vi "Editor Message List Creator.vi"(8 "error in (no error)":errorcluster, 10 "Message List":refnum<vi>, 11 "Hierarchy":refnum<vi>) -> (0 "error out":errorcluster, 3 "Message List Elements":T1[](array[typedef]))   [LabVIEW 2020]
doc: "Create Array of Message List Elements from either the Folder Override or from the Application data folder."
uses:
  Controls/Ctl_MessageListElement.ctl
  Sequencer.lvlib
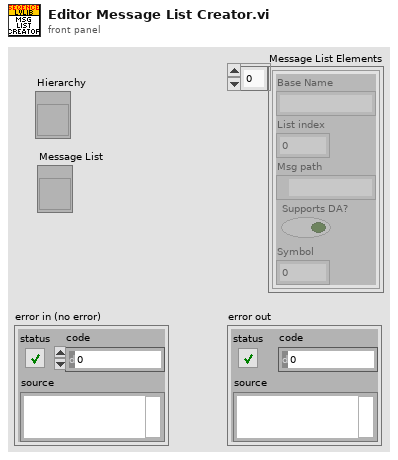
[diagram p1: front panel]
types:
  T1 = typedef "Sequencer.lvlib/Ctl_MessageListElement.ctl" = cluster{"Base Name":string, "List index":i32, "Msg path":path, "Supports DA?":bool, "Symbol":i32}
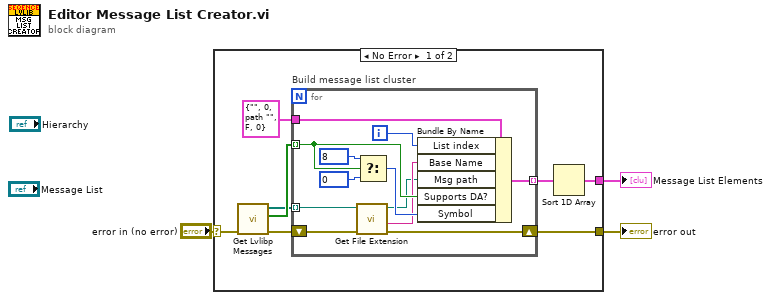
[diagram p0: block diagram]
diagram:
  n1 = case shown="No Error" "error in (no error)" {
    selector: "error in (no error)" -> [w9 w24]
    tunnel: [w10 w24] -> w3
    tunnel: [w8 _] -> w1
    frame No Error {
      n2 = call "Get Lvlibp Messages.vi"("error in (no error)"=w9) -> ("error out"=w11:errorcluster, "Supports Data Access?"=w5:bool[], "Msg Paths"=w4:path[])  [unwired: 7 in, 1 out]
      n3 = for "Build message list cluster" {
        tunnel: w4 -> [w23] mode=indexing
        tunnel: w5 -> [w18] mode=indexing
        shift-right: [w16] -> w10
        shift-left: w11 -> [w20]
        tunnel: T1 {"Base Name"="", "List index"=0, "Msg path"=path "", "Supports DA?"=FALSE, "Symbol"=0} -> [w19]
        tunnel: [w17] -> w7 mode=indexing
        i -> [w14]
        n4 = call <vilib>:"Get File Extension.vi"("error in (no error)"=w20, "file"=w23) -> ("error out"=w16:errorcluster, "filename without extension"=w13:string, "dup file"=w12:path)  [unwired: 5 in, 2 out]
        n5 = Select(t=8, s=w18, f=0) -> (s? t:f=w15:i32)
        n6 = Bundle By Name(cluster=w19, "List index"=w14, "Base Name"=w13, "Msg path"=w12, "Supports DA?"=w18, "Symbol"=w15) -> (w17:T1)
      }
      n7 = Sort 1D Array(array=w7) -> (sorted array=w8:T1[])
    }
    frame Error {
    }
  }
  "error out" <- w3
  "Message List Elements" <- w1
